vi "Generate gRPC Client.vi"(10 "proto file name":string="data_store_service.proto", 11 "source proto directory":path=path "C:/dev/ASW/Source/Protos") -> (0 "error out":errorcluster)   [LabVIEW 2024, in "gRPC Client Generation.lvlib"]
uses:
  gRPC Client Generation.lvlib
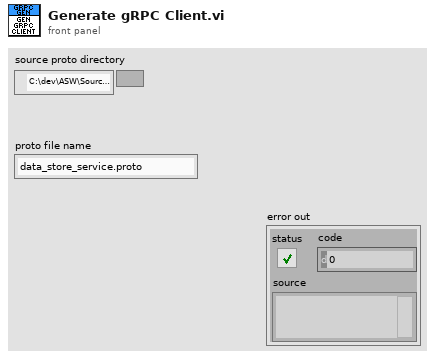
[diagram p1: front panel]
types:
  T1 = typedef "gRPC Client Generation.lvlib/Generation Data.ctl" = cluster{"proto file":path, "imports":path[], "library name":string, "project":path}
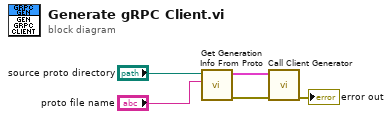
[diagram p0: block diagram]
diagram:
  n1 = call "Get Generation Info From Proto.vi"("proto file name"="proto file name", "source proto directory"="source proto directory") -> ("error out"=w2:errorcluster, "generation data"=w3:T1)  [unwired: 8 in]
  n2 = call "Call Client Generator.vi"("error in"=w2, "generation data"=w3) -> ("error out"=→"error out":errorcluster)  [unwired: 9 in]
